vi "NextState.vi"(0 "object in":refnum<class "PositionTactic.lvclass">, 2 "Robot in":refnum<class "Robot.lvclass">, 4 "GameRef":refnum<data-value>, 5 "error in (no error)":errorcluster) -> (14 "object out":refnum<class "PositionTactic.lvclass">, 19 "error out":errorcluster)   [LabVIEW 2023, in "PositionTactic.lvclass"]
uses:
  PositionTactic.lvclass
  C:/Users/ebert/Documents/codes/SSL/repo/SSL_AI/NewSTP/NewTactics/Tactic_v2_class/Tactic_v2.lvclass
  Robot_class/Robot.lvclass
  Game_class/Game.lvclass
  PositionTactic_states/PositionTactic_states.ctl
  PositionTactic.lvclass/PositionTactic.ctl
panel:
  out "currentState":u8
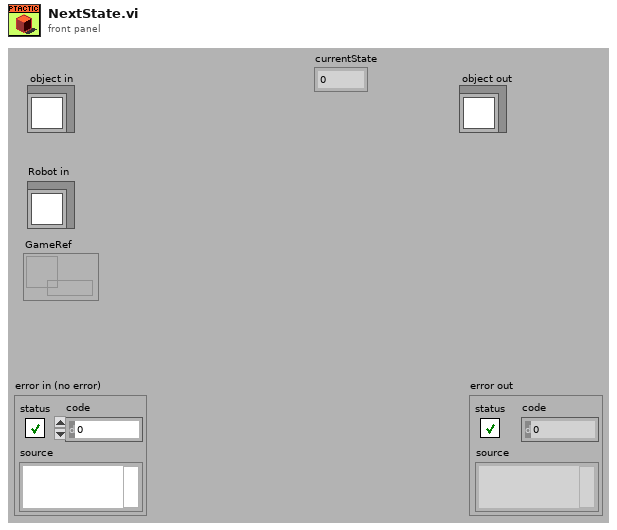
[diagram p1: front panel]
types:
  T1 = typedef "PositionTactic.lvclass/PositionTactic_states.ctl" = enum16{"GoToGuardPosition", "GoToTargetPosition"}
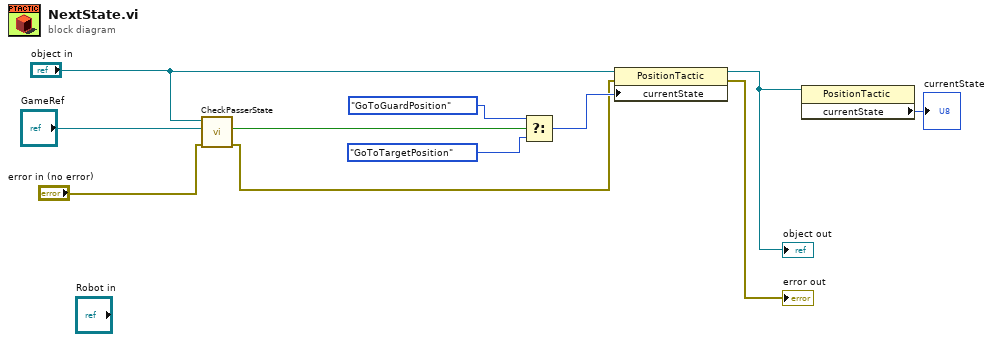
[diagram p0: block diagram]
diagram:
  n1 = call "CheckPasserState.vi"("error in (no error)"="error in (no error)", "GameRef"="GameRef", "object in"="object in") -> ("error out"=w4:errorcluster, "goToGuardPos"=w8:bool)  [unwired: 6 in, 1 out]
  n2 = Select(t=PositionTactic_states."GoToGuardPosition" ("Enum"), s=w8, f=PositionTactic_states."GoToTargetPosition" ("Enum")) -> (s? t:f=w9:T1)
  n3 = property class="PositionTactic"(reference="object in", error in=w4, "currentState"=w9) -> (reference out=w2:refnum<class "PositionTactic.lvclass">, error out=→"error out":errorcluster)
  "object out" <- w2
  n4 = property class="PositionTactic"(reference=w2) -> ("currentState"=→"currentState":u8)  [unwired: 1 in, 2 out]
